vi "Sysdef.SimpleImport.vi"(7 "Overwrite Existing?":bool=TRUE, 8 "error in (no error)":errorcluster, 10 "SysDef":T1 {"Tree"."Properties"."Type" items=["K_STRING", "K_BOOL", "K_I32", "K_U32", "K_DOUBLE", "K_U64", "K_VARIANT", "K_DEPENDENTFILE", "K_DEPENDENTNODE", "K_DATASOURCENODE", "K_U16", "K_DBLARR", "K_U32ARR", "K_I32ARR", "K_STRINGARR", "K_DICTIONARY", "K_DICTIONARYARR"]}, 11 "NodeID":u64) -> (0 "error out":errorcluster, 3 "NodeID out":u64)   [LabVIEW 2015, in "ImportExport.lvlib"]
doc: "Uses the NI VeriStand .NET API. to add or edit the Custom Device Hierarchy (Sections, Channels, Waveforms) as well as its Items Properties using the data from the SysDef cluster."
uses:
  ImportExport.lvlib
  <vilib>/NI/NI VeriStand Advanced SysDef API/_Types/SysDef.Export.ctl
  <vilib>/NI/NI VeriStand Advanced SysDef API/_Types/TreeItem.ctl
  <vilib>/NI/NI VeriStand Advanced SysDef API/_Types/TreeItem.Info.ctl
  <vilib>/NI Veristand/Custom Device API/Custom Device Channel.ctl
  <vilib>/NI Veristand/Custom Device API/Custom Device Channel Type.ctl
  <vilib>/NI Veristand/Custom Device API/Custom Device Waveform.ctl
  <vilib>/NI Veristand/Custom Device API/Custom Device Waveform DataType.ctl
  <vilib>/NI/NI VeriStand Advanced SysDef API/_Types/TreeItem.Property.ctl
  NationalInstruments.VeriStand.SystemDefinitionAPI
  NationalInstruments.VeriStand.SystemStorage
  <vilib>/NI/NI VeriStand Advanced SysDef API/SysDef API/Advanced System Definition.lvlib
  <vilib>/NI Veristand/Custom Device API/Custom Device API.lvlib
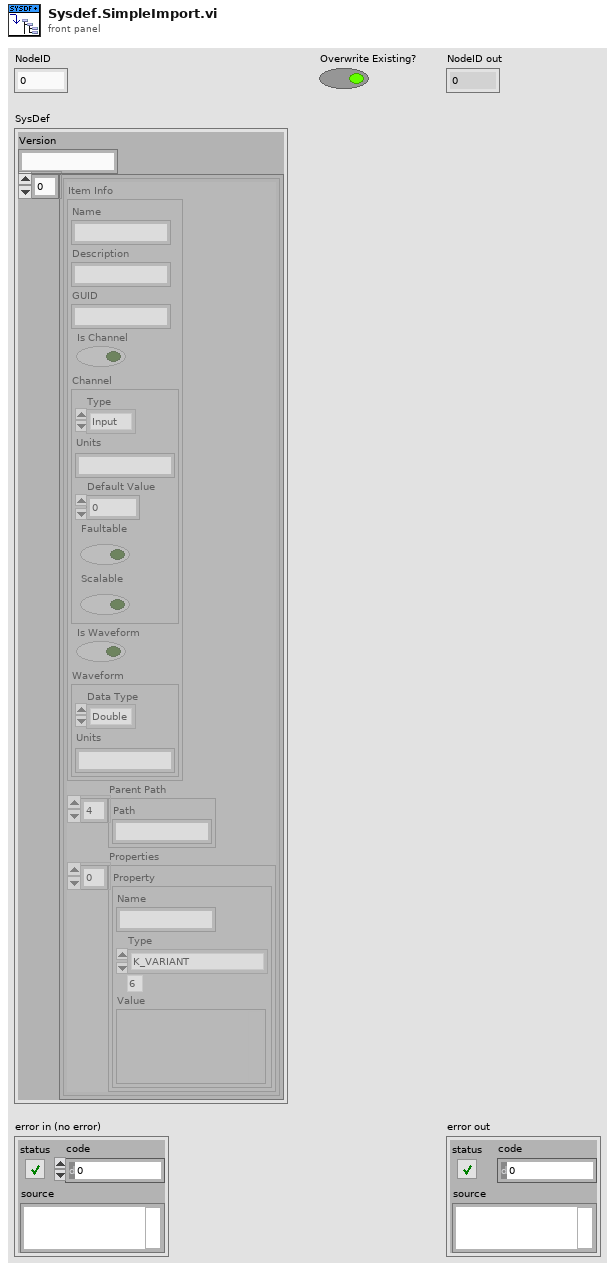
[diagram p1: front panel]
types:
  T1 = typedef "Advanced System Definition.lvlib/SysDef.Export.ctl" = cluster{"Version":string, "Tree":T2[]}
  T2 = typedef "Advanced System Definition.lvlib/TreeItem.ctl" = cluster{"Item Info":T3, "Parent Path":string[], "Properties":T8[]}
  T3 = typedef "Advanced System Definition.lvlib/TreeItem.Info.ctl" = cluster{"Name":string, "Description":string, "GUID":string, "Is Channel":bool, "Channel":T4, "Is Waveform":bool, "Waveform":T6}
  T4 = typedef "Custom Device API.lvlib/Custom Device Channel.ctl" = cluster{"Type":T5, "Units":string, "Default Value":dbl, "Faultable":bool, "Scalable":bool}
  T5 = typedef "Custom Device API.lvlib/Custom Device Channel Type.ctl" = enum16{"Input", "Output"}
  T6 = typedef "Custom Device API.lvlib/Custom Device Waveform.ctl" = cluster{"Data Type":T7, "Units":string}
  T7 = typedef "Custom Device API.lvlib/Custom Device Waveform DataType.ctl" = enum16{"Double", "Complex Double"}
  T8 = typedef "Advanced System Definition.lvlib/TreeItem.Property.ctl" = cluster{"Name":string, "Type":i32, "Value":variant}
  T9 = typedef "Custom Device API.lvlib/Custom Device Item Ref.ctl" = u64
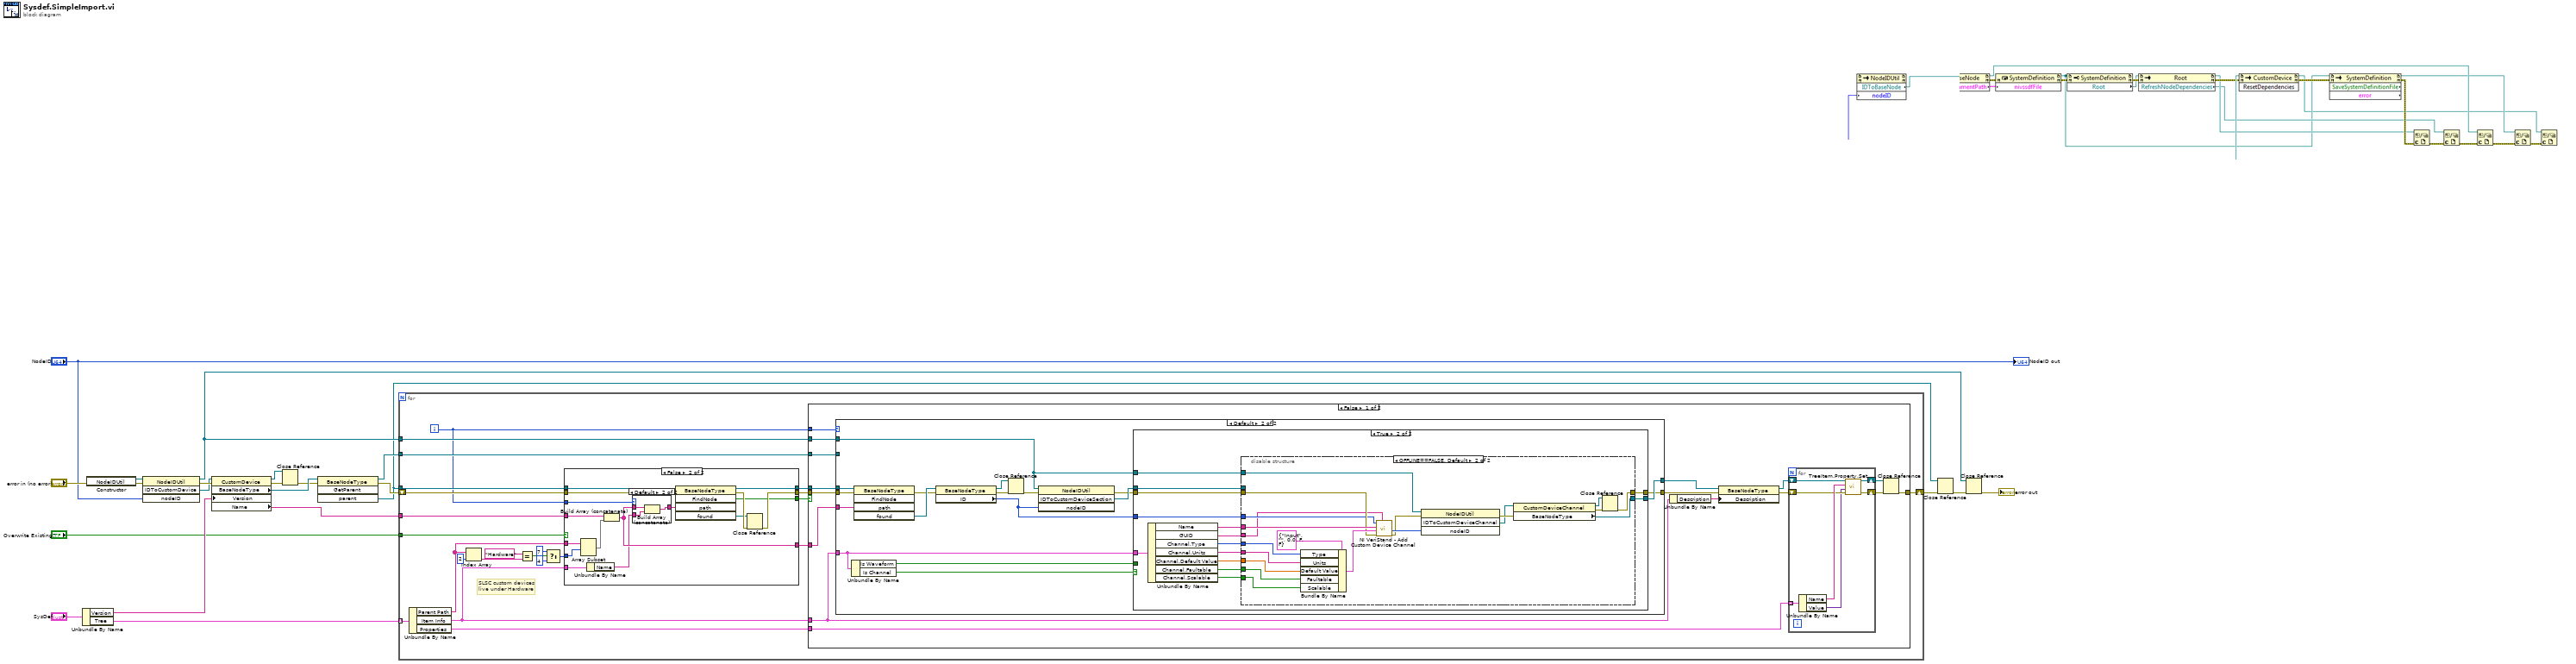
[diagram p0: block diagram]
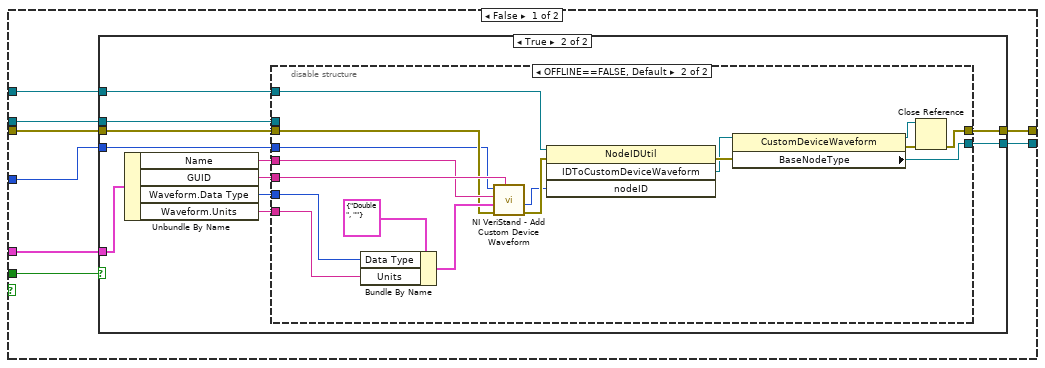
[diagram p3: hidden frame]
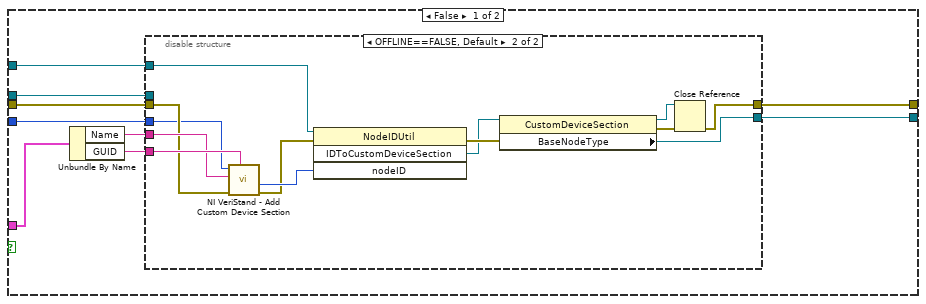
[diagram p4: hidden frame]
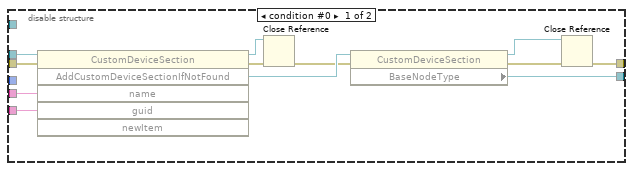
[diagram p5: hidden frame]
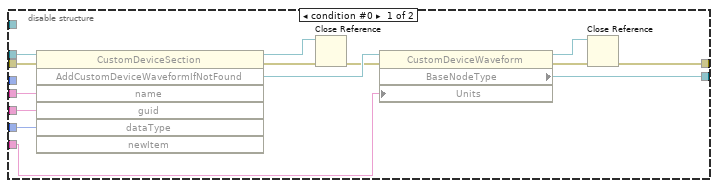
[diagram p6: hidden frame]
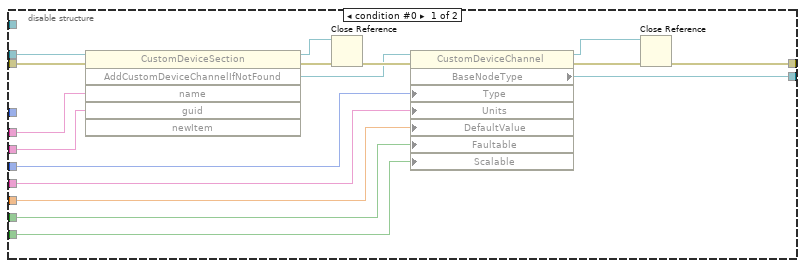
[diagram p7: hidden frame]
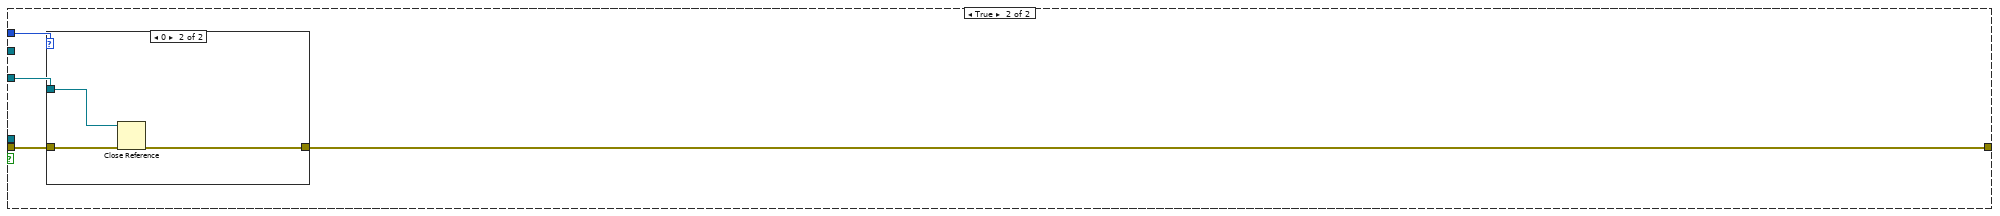
[diagram p8: hidden frame]
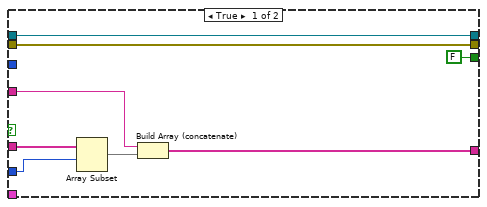
[diagram p10: hidden frame]
diagram:
  n1 = Unbundle By Name("SysDef") -> ("Version"=w20:string, "Tree"=w21:T2[])
  n2 = constructor class="NodeIDUtil"(error in="error in (no error)") -> (reference out=w2:refnum<k24>, error out=w7:errorcluster)  [unwired: 2 in, 1 out]
  n3 = invoke class="NodeIDUtil" method="IDToCustomDevice"(reference=w2, error in=w7, "nodeID"="NodeID") -> (reference out=w13:refnum<k24>, error out=w19:errorcluster, "IDToCustomDevice"=w1:refnum<k24>)  [unwired: 1 in, 1 out]
  n4 = property class="CustomDevice"(reference=w1, error in=w19, "Version"=w20) -> (reference out=w5:refnum<k24>, error out=w4:errorcluster, "BaseNodeType"=w10:refnum<k24>, "Name"=w16:string)
  n5 = Close Reference(reference=w5, error in (no error)=w4) -> (error out=w3:errorcluster)
  n6 = invoke class="BaseNodeType" method="GetParent"(reference=w10, error in=w3) -> (reference out=w17:refnum<k24>, error out=w18:errorcluster, "parent"=w9:refnum<k24>)  [unwired: 2 in, 1 out]
  n7 = for {
    tunnel: w21 -> [w45] mode=indexing
    shift-right: [w43] -> w6
    shift-left: w18 -> [w37]
    tunnel: w17 -> [w42]
    tunnel: w16 -> [w41]
    tunnel: "Overwrite Existing?" -> [w38]
    tunnel: w13 -> [w33]
    tunnel: w9 -> [w32]
    i -> [w31]
    # "SLSC custom devices\nlive under Hardware"
    n8 = Unbundle By Name(w45) -> ("Parent Path"=w30:string[], "Item Info"=w39:T3, "Properties"=w44:T8[])
    n9 = Index Array(array=w30, index=2) -> (element=w28:string)
    n10 = Equal?(x="Hardware", y=w28) -> (x = y?=w26:bool)
    n11 = Select(t=7 ("index"), s=w26, f=4 ("index")) -> (s? t:f=w23:i32)
    n12 = case shown="False" w38 {
      tunnel: w30 -> [w238 w254]
      tunnel: w41 -> [w236 w252]
      tunnel: [w235 w250] -> w40
      tunnel: w39 -> [_ w251]
      tunnel: w37 -> [w233 w248]
      tunnel: w32 -> [w234 w246]
      tunnel: [w234 w240] -> w36
      tunnel: [w233 w244] -> w35
      tunnel: [FALSE ("FindNode") w243] -> w34
      tunnel: w31 -> [_ w242]
      tunnel: w23 -> [w231 w239]
      frame True {
        n13 = Array Subset(array=w238, index=w231) -> (w237:string[])  [unwired: 1 in]
        n14 = Build Array (concatenate)(w236, w237) -> (w235:string[])
      }
      frame False {
        n15 = Array Subset(array=w254, index=w239) -> (w253:string[])  [unwired: 1 in]
        n16 = Unbundle By Name(w251) -> ("Name"=w249:string)
        n17 = Build Array (concatenate)(w252, w253) -> (w250:string[])
        n18 = case shown="Default" w242 {
          tunnel: w250 -> [w255 w258]
          tunnel: w249 -> [_ w257]
          tunnel: [w255 w256] -> w247
          frame 0 {
          }
          frame Default {
            n19 = Build Array (concatenate)(w258, w257) -> (w256:string[])
          }
        }
        n20 = invoke class="BaseNodeType" method="FindNode"(reference=w246, error in=w248, "path"=w247) -> (reference out=w240:refnum<k24>, error out=w245:errorcluster, "FindNode"=w243:bool, "found"=w241:refnum<k24>)  [unwired: 2 in, 1 out]
        n21 = Close Reference(reference=w241, error in (no error)=w245) -> (error out=w244:errorcluster)
      }
    }
    n22 = case shown="False" w34 {
      tunnel: w44 -> [w61 _]
      tunnel: w33 -> [w60 _]
      tunnel: [w57 w223] -> w43
      tunnel: w31 -> [w56 w226]
      tunnel: w42 -> [w55 w224]
      tunnel: w40 -> [w54 _]
      tunnel: w39 -> [w47 _]
      tunnel: w36 -> [w53 _]
      tunnel: w35 -> [w52 w225]
      frame False {
        n23 = case shown="Default" w56 {
          tunnel: w52 -> [w62 w78]
          tunnel: [w62 w70] -> w51
          tunnel: [w63 w71] -> w50
          tunnel: w53 -> [_ w66]
          tunnel: w54 -> [_ w80]
          tunnel: w47 -> [_ w72]
          tunnel: w60 -> [_ w64]
          tunnel: w55 -> [w63 _]
          frame 0 {
          }
          frame Default {
            n24 = Unbundle By Name(w72) -> ("Is Waveform"=w69:bool, "Is Channel"=w73:bool)
            n25 = invoke class="BaseNodeType" method="FindNode"(reference=w66, error in=w78, "path"=w80) -> (error out=w77:errorcluster, "found"=w79:refnum<k24>)  [unwired: 2 in, 3 out]
            n26 = property class="BaseNodeType"(reference=w79, error in=w77) -> (reference out=w67:refnum<k24>, error out=w76:errorcluster, "ID"=w65:u64)
            n27 = Close Reference(reference=w67, error in (no error)=w76) -> (error out=w68:errorcluster)
            n28 = invoke class="NodeIDUtil" method="IDToCustomDeviceSection"(reference=w64, error in=w68, "nodeID"=w65) -> (error out=w74:errorcluster, "IDToCustomDeviceSection"=w75:refnum<k24>)  [unwired: 1 in, 2 out]
            n29 = case shown="True" w73 {
              tunnel: w75 -> [w87 w174]
              tunnel: w74 -> [w86 w171]
              tunnel: w72 -> [w84 w167]
              tunnel: [w85 w170] -> w71
              tunnel: [w83 w168] -> w70
              tunnel: w69 -> [w88 _]
              tunnel: w65 -> [w82 w166]
              tunnel: w64 -> [w81 w165]
              frame False {
                n30 = case shown="True" w88 {
                  tunnel: w87 -> [w96 w133]
                  tunnel: w86 -> [w97 w132]
                  tunnel: [w93 w126] -> w85
                  tunnel: [w92 w128] -> w83
                  tunnel: w84 -> [w95 w131]
                  tunnel: w82 -> [w90 w124]
                  tunnel: w81 -> [w89 w123]
                  frame False {
                    n31 = Unbundle By Name(w95) -> ("Name"=w91:string, "GUID"=w94:string)
                    n32 = disable-structure shown="OFFLINE==FALSE, Default" {
                      disable-tunnel: w97 -> [w107 w120]
                      disable-tunnel: w96 -> [w106 _]
                      disable-tunnel: w94 -> [w105 w122]
                      disable-tunnel: [w103 w111] -> w93
                      disable-tunnel: [w99 w110] -> w92
                      disable-tunnel: w91 -> [w98 w121]
                      disable-tunnel: w90 -> [_ w119]
                      disable-tunnel: w89 -> [_ w112]
                      frame condition #0 {
                        n33 = invoke class="CustomDeviceSection" method="AddCustomDeviceSectionIfNotFound"(reference=w106, error in=w107, "name"=w98, "guid"=w105) -> (reference out=w108:refnum<k24>, error out=w109:errorcluster, "AddCustomDeviceSectionIfNotFound"=w104:refnum<k24>)  [unwired: 2 in, 3 out]
                        n34 = Close Reference(reference=w108, error in (no error)=w109) -> (error out=w102:errorcluster)
                        n35 = property class="CustomDeviceSection"(reference=w104, error in=w102) -> (reference out=w101:refnum<k24>, error out=w100:errorcluster, "BaseNodeType"=w103:refnum<k24>)
                        n36 = Close Reference(reference=w101, error in (no error)=w100) -> (error out=w99:errorcluster)
                      }
                      frame condition #1 (active) {
                        n37 = call <vilib>:"NI VeriStand - Add Custom Device Section.vi"("GUID (Default Section)"=w122, "error in (no error)"=w120, "Section Name"=w121, "Parent Ref in"=w119) -> ("error out"=w113:errorcluster, "Section Ptr"=w114:T9)  [unwired: 4 in, 2 out]
                        n38 = invoke class="NodeIDUtil" method="IDToCustomDeviceSection"(reference=w112, error in=w113, "nodeID"=w114) -> (error out=w118:errorcluster, "IDToCustomDeviceSection"=w117:refnum<k24>)  [unwired: 1 in, 2 out]
                        n39 = property class="CustomDeviceSection"(reference=w117, error in=w118) -> (reference out=w116:refnum<k24>, error out=w115:errorcluster, "BaseNodeType"=w111:refnum<k24>)
                        n40 = Close Reference(reference=w116, error in (no error)=w115) -> (error out=w110:errorcluster)
                      }
                    }
                  }
                  frame True {
                    n41 = Unbundle By Name(w131) -> ("Name"=w125:string, "GUID"=w130:string, "Waveform.Data Type"=w129:T7, "Waveform.Units"=w127:string)
                    n42 = disable-structure shown="OFFLINE==FALSE, Default" {
                      disable-tunnel: w133 -> [w143 _]
                      disable-tunnel: w132 -> [w142 w158]
                      disable-tunnel: w130 -> [w141 w164]
                      disable-tunnel: w129 -> [w140 w162]
                      disable-tunnel: [w137 w152] -> w128
                      disable-tunnel: w127 -> [w136 w161]
                      disable-tunnel: [w135 w151] -> w126
                      disable-tunnel: w125 -> [w134 w159]
                      disable-tunnel: w124 -> [_ w149]
                      disable-tunnel: w123 -> [_ w148]
                      frame condition #0 {
                        n43 = invoke class="CustomDeviceSection" method="AddCustomDeviceWaveformIfNotFound"(reference=w143, error in=w142, "name"=w134, "guid"=w141, "dataType"=w140) -> (reference out=w146:refnum<k24>, error out=w147:errorcluster, "AddCustomDeviceWaveformIfNotFound"=w145:refnum<k24>)  [unwired: 2 in, 4 out]
                        n44 = Close Reference(reference=w146, error in (no error)=w147) -> (error out=w144:errorcluster)
                        n45 = property class="CustomDeviceWaveform"(reference=w145, error in=w144, "Units"=w136) -> (reference out=w139:refnum<k24>, error out=w138:errorcluster, "BaseNodeType"=w135:refnum<k24>)
                        n46 = Close Reference(reference=w139, error in (no error)=w138) -> (error out=w137:errorcluster)
                      }
                      frame condition #1 (active) {
                        n47 = Bundle By Name(cluster=T6 {"Data Type"=enum."Double", "Units"=""} ("Waveform"), "Data Type"=w162, "Units"=w161) -> (w160:T6)
                        n48 = call <vilib>:"NI VeriStand - Add Custom Device Waveform.vi"("GUID (Default Waveform)"=w164, "error in (no error)"=w158, "Waveform"=w160, "Waveform Name"=w159, "Parent Ref in"=w149) -> ("error out"=w153:errorcluster, "Waveform Ref"=w150:T9)  [unwired: 3 in, 2 out]
                        n49 = invoke class="NodeIDUtil" method="IDToCustomDeviceWaveform"(reference=w148, error in=w153, "nodeID"=w150) -> (error out=w157:errorcluster, "IDToCustomDeviceWaveform"=w156:refnum<k24>)  [unwired: 1 in, 2 out]
                        n50 = property class="CustomDeviceWaveform"(reference=w156, error in=w157) -> (reference out=w155:refnum<k24>, error out=w154:errorcluster, "BaseNodeType"=w151:refnum<k24>)
                        n51 = Close Reference(reference=w155, error in (no error)=w154) -> (error out=w152:errorcluster)
                      }
                    }
                  }
                }
              }
              frame True {
                n52 = Unbundle By Name(w167) -> ("Name"=w169:string, "GUID"=w173:string, "Channel.Type"=w172:T5, "Channel.Units"=w178:string, "Channel.Default Value"=w177:dbl, "Channel.Faultable"=w176:bool, "Channel.Scalable"=w175:bool)
                n53 = disable-structure shown="OFFLINE==FALSE, Default" {
                  disable-tunnel: w178 -> [w194 w212]
                  disable-tunnel: w177 -> [w193 w211]
                  disable-tunnel: w176 -> [w192 w210]
                  disable-tunnel: w175 -> [w191 w209]
                  disable-tunnel: w174 -> [w190 _]
                  disable-tunnel: w173 -> [w189 w196]
                  disable-tunnel: w172 -> [w188 w213]
                  disable-tunnel: w171 -> [w186 w207]
                  disable-tunnel: [w185 w203] -> w170
                  disable-tunnel: w169 -> [w184 w215]
                  disable-tunnel: [w183 w197] -> w168
                  disable-tunnel: w166 -> [_ w206]
                  disable-tunnel: w165 -> [_ w204]
                  frame condition #0 {
                    n54 = invoke class="CustomDeviceSection" method="AddCustomDeviceChannelIfNotFound"(reference=w190, error in=w186, "name"=w184, "guid"=w189) -> (reference out=w179:refnum<k24>, error out=w182:errorcluster, "AddCustomDeviceChannelIfNotFound"=w180:refnum<k24>)  [unwired: 2 in, 3 out]
                    n55 = Close Reference(reference=w179, error in (no error)=w182) -> (error out=w195:errorcluster)
                    n56 = property class="CustomDeviceChannel"(reference=w180, error in=w195, "Type"=w188, "Units"=w194, "DefaultValue"=w193, "Faultable"=w192, "Scalable"=w191) -> (reference out=w187:refnum<k24>, error out=w181:errorcluster, "BaseNodeType"=w185:refnum<k24>)
                    n57 = Close Reference(reference=w187, error in (no error)=w181) -> (error out=w183:errorcluster)
                  }
                  frame condition #1 (active) {
                    n58 = Bundle By Name(cluster=T4 {"Type"=enum."Input", "Units"="", "Default Value"=0.0, "Faultable"=FALSE, "Scalable"=FALSE} ("Channel"), "Type"=w213, "Units"=w212, "Default Value"=w211, "Faultable"=w210, "Scalable"=w209) -> (w208:T4)
                    n59 = call <vilib>:"NI VeriStand - Add Custom Device Channel.vi"("GUID (Default Channel)"=w196, "error in (no error)"=w207, "Channel"=w208, "Channel Name"=w215, "Parent Ref in"=w206) -> ("error out"=w202:errorcluster, "Channel Ref"=w205:T9)  [unwired: 3 in, 2 out]
                    n60 = invoke class="NodeIDUtil" method="IDToCustomDeviceChannel"(reference=w204, error in=w202, "nodeID"=w205) -> (error out=w201:errorcluster, "IDToCustomDeviceChannel"=w200:refnum<k24>)  [unwired: 1 in, 2 out]
                    n61 = property class="CustomDeviceChannel"(reference=w200, error in=w201) -> (reference out=w199:refnum<k24>, error out=w198:errorcluster, "BaseNodeType"=w203:refnum<k24>)
                    n62 = Close Reference(reference=w199, error in (no error)=w198) -> (error out=w197:errorcluster)
                  }
                }
              }
            }
          }
        }
        n63 = Unbundle By Name(w47) -> ("Description"=w46:string)
        n64 = property class="BaseNodeType"(reference=w50, error in=w51, "Description"=w46) -> (reference out=w48:refnum<k24>, error out=w49:errorcluster)
        n65 = for {
          shift-right: [w222] -> w58
          shift-left: w49 -> [w217]
          tunnel: w61 -> [w220] mode=indexing
          shift-right: [w219] -> w59
          shift-left: w48 -> [w221]
          n66 = Unbundle By Name(w220) -> ("Name"=w218:string, "Value"=w216:variant)
          n67 = call <vilib>:"TreeItem.Property.Set.vi"("error in (no error)"=w217, "Value"=w216, "Property Name"=w218, "BaseNodeType"=w221) -> ("error out"=w222:errorcluster, "BaseNodeType"=w219:refnum<k24>)  [unwired: 5 in, 1 out]
        }
        n68 = Close Reference(reference=w59, error in (no error)=w58) -> (error out=w57:errorcluster)
      }
      frame True {
        n69 = case shown="0" w226 {
          tunnel: w225 -> [w227 w230]
          tunnel: [w227 w229] -> w223
          tunnel: w224 -> [_ w228]
          frame Default {
          }
          frame 0 {
            n70 = Close Reference(reference=w228, error in (no error)=w230) -> (error out=w229:errorcluster)
          }
        }
      }
    }
  }
  n71 = Close Reference(reference=w9, error in (no error)=w6) -> (error out=w14:errorcluster)
  n72 = Close Reference(reference=w13, error in (no error)=w14) -> (error out=→"error out":errorcluster)
  "NodeID out" <- "NodeID"
